vi "S2C_BldDeleteEntry.vi"(8 "Error In":errorcluster, 11 "VKey":T1) -> (0 "Error Out":errorcluster)   [LabVIEW 2015]
doc: "Deletes the selected items from the script table."
uses:
  <vilib>/event_ctls.llb/eventvkey.ctl
  Globals/S2C_Globals.vi
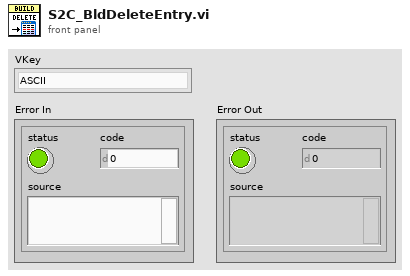
[diagram p1: front panel]
types:
  T1 = typedef "eventvkey.ctl" = enum16{"ASCII", "Enter", "Return", "Shift", "Ctrl", "Alt", "Cmd", "Opt", "Caps", "NumLock", "Clear", "Break", "Up", "Down", "Left", "Right", "Insert", "Delete", "Home", "End", "PageUp", "PageDown", "Escape", "Help", "Pause", "ScrollLock", "F1", "F2", "F3", "F4", "F5", "F6", "F7", "F8", "F9", "F10", "F11", "F12", "F13", "F14", "F15", "F16", "F17", "F18", "F19", "F20", "F21", "F22", "F23", "F24", "Play", "VolumeUp", "VolumeDown", "Mute", "Two Byte Char"}
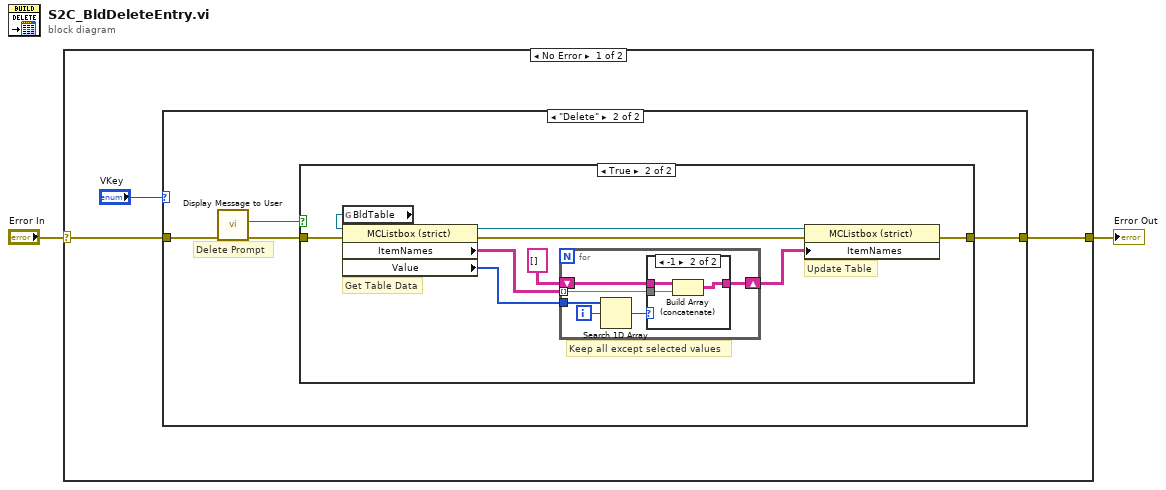
[diagram p0: block diagram]
diagram:
  n1 = case shown="No Error" "Error In" {
    selector: "Error In" -> [w4 w31]
    tunnel: [w5 w31] -> w1
    frame No Error {
      n2 = case shown="\"Delete\"" "VKey" {
        tunnel: [w6 w8] -> w5
        tunnel: w4 -> [w6 w7]
        frame "ASCII", Default {
          # "This VI is only designed to handle the \"Delete\" request"
        }
        frame "Delete" {
          # "Delete Prompt"
          n3 = call "Display Message to User"("error in (no error)"=w7) -> ("error out"=w9:errorcluster, "Delete"=w10:bool)  [unwired: 9 in]
          n4 = case shown="True" w10 {
            tunnel: w9 -> [w11 w20]
            tunnel: [w11 w19] -> w8
            frame False {
              # "Delete operation cancelled by user"
            }
            frame True {
              # "Keep all except selected values"
              # "Update Table"
              # "Get Table Data"
              n5 = global read "S2C_Globals.vi" "BldTable"() -> (w18:refnum<vi>)
              n6 = property on="Property Node" class="MCListbox (strict)"(reference=w18, error in=w20) -> (reference out=w16:refnum<vi>, error out=w17:errorcluster, "ItemNames"=w14:string[][], "Value"=w15:i32[])
              n7 = for {
                tunnel: w14 -> [w22] mode=indexing
                tunnel: w15 -> [w26]
                shift-right: [w21] -> w12
                shift-left: string[][] [] ("Item Names") -> [w23]
                i -> [w25]
                n8 = Search 1D Array(1D array=w26, element=w25) -> (index of element=w24:i32)  [unwired: 1 in]
                n9 = case shown="-1" w24 {
                  tunnel: w23 -> [w27 w30]
                  tunnel: w22 -> [_ w29]
                  tunnel: [w27 w28] -> w21
                  frame 0, Default {
                  }
                  frame -1 {
                    n10 = Build Array (concatenate)(w30, w29) -> (w28:string[][])
                  }
                }
              }
              n11 = property on="Property Node" class="MCListbox (strict)"(reference=w16, error in=w17, "ItemNames"=w12) -> (error out=w19:errorcluster)  [unwired: 1 out]
            }
          }
        }
      }
    }
    frame Error {
    }
  }
  "Error Out" <- w1
